vi "Global_KeyDown.vi"() -> ()   [LabVIEW 2021]
uses:
  TypeDef/KeyDown.ctl
panel:
  in  "Key down":T1
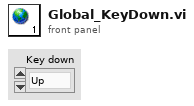
[diagram p1: front panel]
types:
  T1 = typedef "KeyDown.ctl" = enum16{"Up", "Down", "Left", "Right"}
diagram:
